vi "SetSpeed100RPM BROOKFIELD.vi"() -> ()   [LabVIEW 2019]
uses:
  <vilib>/Instr/_visa.llb/VISA Configure Serial Port (Instr).vi
panel:
  out "Control Circuitry Enabled":bool
  out "Motor On":bool
  out "Motor Stopped":bool
  out "Auto-zero Complete":bool
  out "Motor Circuit Error":bool
  out "Diagnostics Error":bool
  out "Invalid Command Received":bool
  out "Torque% Offset":dbl
  in  "rpm setpoint":i32
  in  "Stop Motor":bool
  in  "nnn rpm":bool
  in  "zero":bool
  in  "enable":bool
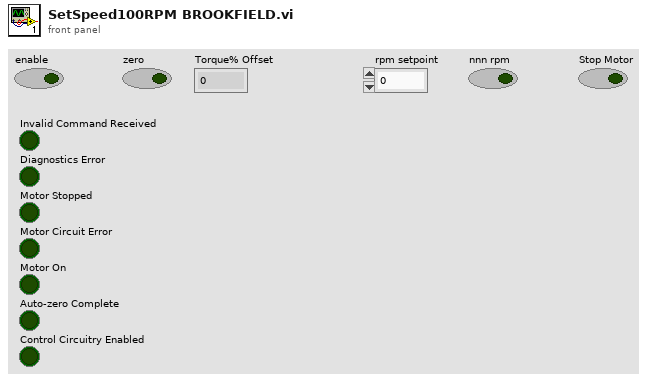
[diagram p1: front panel]
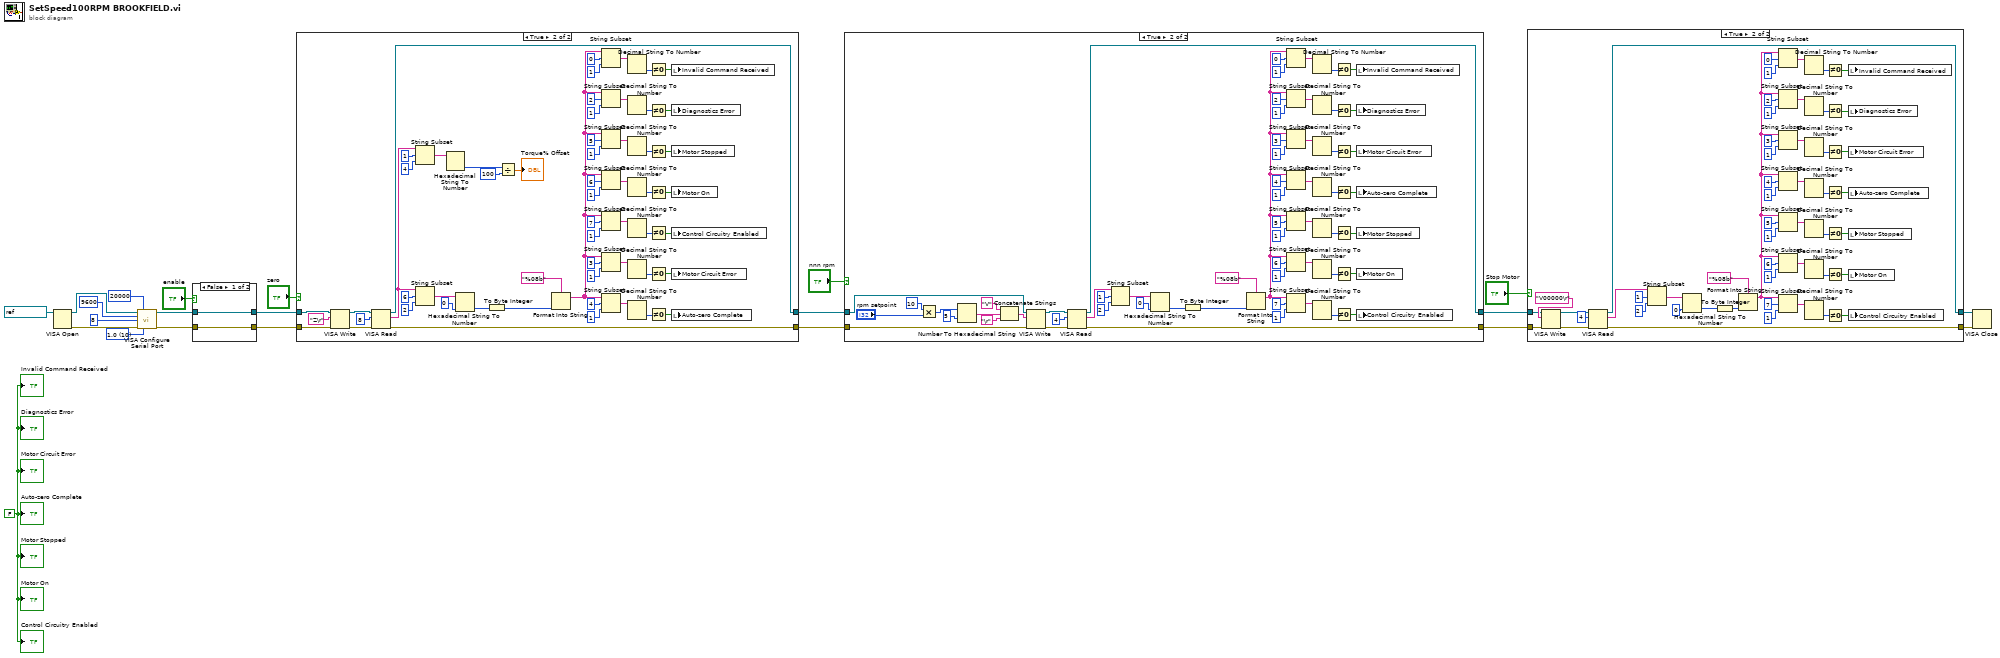
[diagram p0: block diagram]
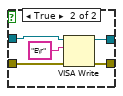
[diagram p5: hidden frame]
diagram:
  w2 = FALSE
  w16 = u16 10 items=["1.0"=10, "1.5"=15, "2.0"=20] ("stop bits (10: 1 bit)")
  n1 = VISA Open(VISA resource name=refnum<visa-resource-name> "COM11" ("Conductivity Port")) -> (VISA resource name=w20:refnum<visa-resource-name>, error out=w22:errorcluster)  [unwired: 4 in]
  n2 = call-poly "VISA Configure Serial Port"("VISA resource name"=w20, "timeout (10sec)"=u32 20000, "baud rate (9600)"=u32 9600, "data bits (8)"=u16 8, "error in (no error)"=w22, "stop bits (10: 1 bit)"=w16) -> ("VISA resource name out"=w15:refnum<visa-resource-name>, "error out"=w10:errorcluster)  [unwired: 8 in]
  n3 = case shown="False" "enable" {
    tunnel: w15 -> [w24 w29]
    tunnel: [w24 w28] -> w14
    tunnel: [w23 w27] -> w11
    tunnel: w10 -> [w23 w26]
    frame False {
    }
    frame True {
      n4 = VISA Write(VISA resource name=w29, write buffer="E\r", error in (no error)=w26) -> (VISA resource name out=w28:refnum<visa-resource-name>, error out=w27:errorcluster)  [unwired: 1 out]
    }
  }
  n5 = case shown="True" "zero" {
    tunnel: w14 -> [w31 w89]
    tunnel: [w31 w84] -> w13
    tunnel: [w30 w83] -> w12
    tunnel: w11 -> [w30 w88]
    frame False {
    }
    frame True {
      n6 = VISA Write(VISA resource name=w89, write buffer="Z\r", error in (no error)=w88) -> (VISA resource name out=w85:refnum<visa-resource-name>, error out=w82:errorcluster)  [unwired: 1 out]
      n7 = VISA Read(VISA resource name=w85, byte count=u32 8, error in (no error)=w82) -> (VISA resource name out=w84:refnum<visa-resource-name>, read buffer=w39:string, error out=w83:errorcluster)  [unwired: 1 out]
      n8 = String Subset(string=w39, offset (0)=1, length (rest)=4 ("length (rest)")) -> (substring=w79:string)
      n9 = String Subset(string=w39, offset (0)=6, length (rest)=2 ("length (rest)")) -> (substring=w73:string)
      n10 = Hexadecimal String To Number(string=w79) -> (number=w78:u32)  [unwired: 2 in, 1 out]
      n11 = Hexadecimal String To Number(string=w73, default (0uL)=u32 0 ("default (0 U32)")) -> (number=w65:u32)  [unwired: 1 in, 1 out]
      n12 = To Byte Integer(number=w65) -> (8bit integer=w66:i8)
      n13 = Divide(x=w78, y=u32 100) -> (x/y=→"Torque% Offset":dbl)
      n14 = Format Into String(format string="%08b", w66) -> (resulting string=w40:string)  [unwired: 2 in, 1 out]
      n15 = String Subset(string=w40, offset (0)=0, length (rest)=1 ("length (rest)")) -> (substring=w69:string)
      n16 = String Subset(string=w40, offset (0)=2, length (rest)=1 ("length (rest)")) -> (substring=w63:string)
      n17 = String Subset(string=w40, offset (0)=5, length (rest)=1 ("length (rest)")) -> (substring=w50:string)
      n18 = String Subset(string=w40, offset (0)=6, length (rest)=1 ("length (rest)")) -> (substring=w47:string)
      n19 = String Subset(string=w40, offset (0)=7, length (rest)=1 ("length (rest)")) -> (substring=w42:string)
      n20 = String Subset(string=w40, offset (0)=3, length (rest)=1 ("length (rest)")) -> (substring=w58:string)
      n21 = String Subset(string=w40, offset (0)=4, length (rest)=1 ("length (rest)")) -> (substring=w55:string)
      n22 = Decimal String To Number(string=w69) -> (number=w68:i32)  [unwired: 2 in, 1 out]
      n23 = Decimal String To Number(string=w63) -> (number=w64:i32)  [unwired: 2 in, 1 out]
      n24 = Decimal String To Number(string=w50) -> (number=w49:i32)  [unwired: 2 in, 1 out]
      n25 = Decimal String To Number(string=w47) -> (number=w48:i32)  [unwired: 2 in, 1 out]
      n26 = Decimal String To Number(string=w42) -> (number=w41:i32)  [unwired: 2 in, 1 out]
      n27 = Decimal String To Number(string=w58) -> (number=w57:i32)  [unwired: 2 in, 1 out]
      n28 = Decimal String To Number(string=w55) -> (number=w56:i32)  [unwired: 2 in, 1 out]
      n29 = Not Equal To 0?(x=w68) -> (x != 0?=w32:bool)
      n30 = Not Equal To 0?(x=w64) -> (x != 0?=w33:bool)
      n31 = Not Equal To 0?(x=w49) -> (x != 0?=w36:bool)
      n32 = Not Equal To 0?(x=w48) -> (x != 0?=w37:bool)
      n33 = Not Equal To 0?(x=w41) -> (x != 0?=w38:bool)
      n34 = Not Equal To 0?(x=w57) -> (x != 0?=w34:bool)
      n35 = Not Equal To 0?(x=w56) -> (x != 0?=w35:bool)
      n36 = local write "Invalid Command Received"(w32) -> ()
      n37 = local write "Diagnostics Error"(w33) -> ()
      n38 = local write "Motor Stopped"(w36) -> ()
      n39 = local write "Motor On"(w37) -> ()
      n40 = local write "Control Circuitry Enabled"(w38) -> ()
      n41 = local write "Motor Circuit Error"(w34) -> ()
      n42 = local write "Auto-zero Complete"(w35) -> ()
    }
  }
  n43 = case shown="True" "nnn rpm" {
    tunnel: w13 -> [w91 w150]
    tunnel: w12 -> [w90 w149]
    tunnel: [w90 w136] -> w6
    tunnel: [w91 w137] -> w5
    frame False {
    }
    frame True {
      n44 = Multiply(x=10, y="rpm setpoint") -> (x*y=w145:i32)
      n45 = Number To Hexadecimal String(1:i16 5 ("width (-)"), 2:w145) -> (0:w143:string)
      n46 = Concatenate Strings("V" ("string"), w143, "\r") -> (w141:string)
      n47 = VISA Write(VISA resource name=w150, write buffer=w141, error in (no error)=w149) -> (VISA resource name out=w140:refnum<visa-resource-name>, error out=w139:errorcluster)  [unwired: 1 out]
      n48 = VISA Read(VISA resource name=w140, byte count=u32 4, error in (no error)=w139) -> (VISA resource name out=w137:refnum<visa-resource-name>, read buffer=w92:string, error out=w136:errorcluster)  [unwired: 1 out]
      n49 = String Subset(string=w92, offset (0)=1, length (rest)=2 ("length (rest)")) -> (substring=w102:string)
      n50 = Hexadecimal String To Number(string=w102, default (0uL)=u32 0 ("default (0 U32)")) -> (number=w110:u32)  [unwired: 1 in, 1 out]
      n51 = To Byte Integer(number=w110) -> (8bit integer=w109:i8)
      n52 = Format Into String(format string="%08b", w109) -> (resulting string=w135:string)  [unwired: 2 in, 1 out]
      n53 = String Subset(string=w135, offset (0)=0, length (rest)=1 ("length (rest)")) -> (substring=w106:string)
      n54 = String Subset(string=w135, offset (0)=2, length (rest)=1 ("length (rest)")) -> (substring=w112:string)
      n55 = String Subset(string=w135, offset (0)=3, length (rest)=1 ("length (rest)")) -> (substring=w117:string)
      n56 = String Subset(string=w135, offset (0)=4, length (rest)=1 ("length (rest)")) -> (substring=w120:string)
      n57 = String Subset(string=w135, offset (0)=5, length (rest)=1 ("length (rest)")) -> (substring=w125:string)
      n58 = String Subset(string=w135, offset (0)=6, length (rest)=1 ("length (rest)")) -> (substring=w128:string)
      n59 = String Subset(string=w135, offset (0)=7, length (rest)=1 ("length (rest)")) -> (substring=w133:string)
      n60 = Decimal String To Number(string=w106) -> (number=w107:i32)  [unwired: 2 in, 1 out]
      n61 = Decimal String To Number(string=w112) -> (number=w111:i32)  [unwired: 2 in, 1 out]
      n62 = Decimal String To Number(string=w117) -> (number=w118:i32)  [unwired: 2 in, 1 out]
      n63 = Decimal String To Number(string=w120) -> (number=w119:i32)  [unwired: 2 in, 1 out]
      n64 = Decimal String To Number(string=w125) -> (number=w126:i32)  [unwired: 2 in, 1 out]
      n65 = Decimal String To Number(string=w128) -> (number=w127:i32)  [unwired: 2 in, 1 out]
      n66 = Decimal String To Number(string=w133) -> (number=w134:i32)  [unwired: 2 in, 1 out]
      n67 = Not Equal To 0?(x=w107) -> (x != 0?=w99:bool)
      n68 = Not Equal To 0?(x=w111) -> (x != 0?=w98:bool)
      n69 = Not Equal To 0?(x=w118) -> (x != 0?=w97:bool)
      n70 = Not Equal To 0?(x=w119) -> (x != 0?=w96:bool)
      n71 = Not Equal To 0?(x=w126) -> (x != 0?=w95:bool)
      n72 = Not Equal To 0?(x=w127) -> (x != 0?=w94:bool)
      n73 = Not Equal To 0?(x=w134) -> (x != 0?=w93:bool)
      n74 = local write "Invalid Command Received"(w99) -> ()
      n75 = local write "Diagnostics Error"(w98) -> ()
      n76 = local write "Motor Circuit Error"(w97) -> ()
      n77 = local write "Auto-zero Complete"(w96) -> ()
      n78 = local write "Motor Stopped"(w95) -> ()
      n79 = local write "Motor On"(w94) -> ()
      n80 = local write "Control Circuitry Enabled"(w93) -> ()
    }
  }
  n81 = case shown="True" "Stop Motor" {
    tunnel: w6 -> [w152 w203]
    tunnel: [w151 w154] -> w4
    tunnel: w5 -> [w151 w202]
    tunnel: [w152 w153] -> w1
    frame False {
    }
    frame True {
      n82 = VISA Write(VISA resource name=w202, write buffer="V00000\r", error in (no error)=w203) -> (VISA resource name out=w155:refnum<visa-resource-name>, error out=w156:errorcluster)  [unwired: 1 out]
      n83 = VISA Read(VISA resource name=w155, byte count=u32 4, error in (no error)=w156) -> (VISA resource name out=w154:refnum<visa-resource-name>, read buffer=w201:string, error out=w153:errorcluster)  [unwired: 1 out]
      n84 = String Subset(string=w201, offset (0)=1, length (rest)=2 ("length (rest)")) -> (substring=w191:string)
      n85 = Hexadecimal String To Number(string=w191, default (0uL)=u32 0 ("default (0 U32)")) -> (number=w183:u32)  [unwired: 1 in, 1 out]
      n86 = To Byte Integer(number=w183) -> (8bit integer=w184:i8)
      n87 = Format Into String(format string="%08b", w184) -> (resulting string=w158:string)  [unwired: 2 in, 1 out]
      n88 = String Subset(string=w158, offset (0)=0, length (rest)=1 ("length (rest)")) -> (substring=w187:string)
      n89 = String Subset(string=w158, offset (0)=2, length (rest)=1 ("length (rest)")) -> (substring=w181:string)
      n90 = String Subset(string=w158, offset (0)=3, length (rest)=1 ("length (rest)")) -> (substring=w176:string)
      n91 = String Subset(string=w158, offset (0)=4, length (rest)=1 ("length (rest)")) -> (substring=w173:string)
      n92 = String Subset(string=w158, offset (0)=5, length (rest)=1 ("length (rest)")) -> (substring=w168:string)
      n93 = String Subset(string=w158, offset (0)=6, length (rest)=1 ("length (rest)")) -> (substring=w165:string)
      n94 = String Subset(string=w158, offset (0)=7, length (rest)=1 ("length (rest)")) -> (substring=w160:string)
      n95 = Decimal String To Number(string=w187) -> (number=w186:i32)  [unwired: 2 in, 1 out]
      n96 = Decimal String To Number(string=w181) -> (number=w182:i32)  [unwired: 2 in, 1 out]
      n97 = Decimal String To Number(string=w176) -> (number=w175:i32)  [unwired: 2 in, 1 out]
      n98 = Decimal String To Number(string=w173) -> (number=w174:i32)  [unwired: 2 in, 1 out]
      n99 = Decimal String To Number(string=w168) -> (number=w167:i32)  [unwired: 2 in, 1 out]
      n100 = Decimal String To Number(string=w165) -> (number=w166:i32)  [unwired: 2 in, 1 out]
      n101 = Decimal String To Number(string=w160) -> (number=w159:i32)  [unwired: 2 in, 1 out]
      n102 = Not Equal To 0?(x=w186) -> (x != 0?=w194:bool)
      n103 = Not Equal To 0?(x=w182) -> (x != 0?=w195:bool)
      n104 = Not Equal To 0?(x=w175) -> (x != 0?=w196:bool)
      n105 = Not Equal To 0?(x=w174) -> (x != 0?=w197:bool)
      n106 = Not Equal To 0?(x=w167) -> (x != 0?=w198:bool)
      n107 = Not Equal To 0?(x=w166) -> (x != 0?=w199:bool)
      n108 = Not Equal To 0?(x=w159) -> (x != 0?=w200:bool)
      n109 = local write "Invalid Command Received"(w194) -> ()
      n110 = local write "Diagnostics Error"(w195) -> ()
      n111 = local write "Motor Circuit Error"(w196) -> ()
      n112 = local write "Auto-zero Complete"(w197) -> ()
      n113 = local write "Motor Stopped"(w198) -> ()
      n114 = local write "Motor On"(w199) -> ()
      n115 = local write "Control Circuitry Enabled"(w200) -> ()
    }
  }
  n116 = VISA Close(VISA resource name=w4, error in (no error)=w1) -> ()  [unwired: 1 out]
  "Invalid Command Received" <- w2
  "Diagnostics Error" <- w2
  "Motor Circuit Error" <- w2
  "Auto-zero Complete" <- w2
  "Motor Stopped" <- w2
  "Motor On" <- w2
  "Control Circuitry Enabled" <- w2
